vi "alum dose a+ b(HFTurbidity)0.5.vi"(4 "State":i16, 5 "Time":dbl format="%.2f", 6 "Sensor Values":dbl[](array[numeric]), 7 "Set Points":dbl[](array[numeric])) -> (0 "required data":T1={"Set Point names"=["a", "b", "raw water turbidity"], "required number of setpoints"=3, "required number of sensors"=0, "Sensor names"=[""]}, 3 "fraction on":dbl)   [LabVIEW 2010]
panel:
  # "Enter the correct information for this control code in the required data structure below. Then make the current value default by right clicking on the border of the data structure."
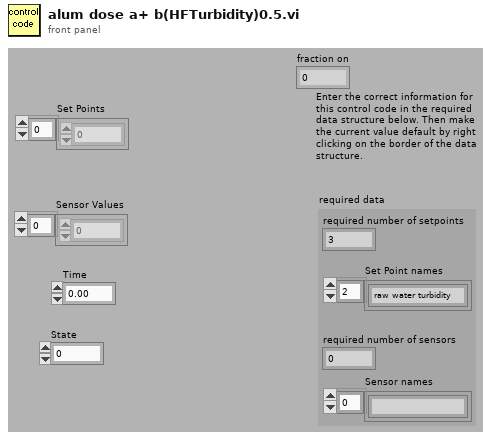
[diagram p1: front panel]
types:
  T1 = cluster{"Set Point names":string[], "required number of setpoints":u8, "required number of sensors":u8, "Sensor names":string[]}
  T2 = cluster{"Set Points[0]":dbl, "Set Points[1]":dbl, "Set Points[2]":dbl}
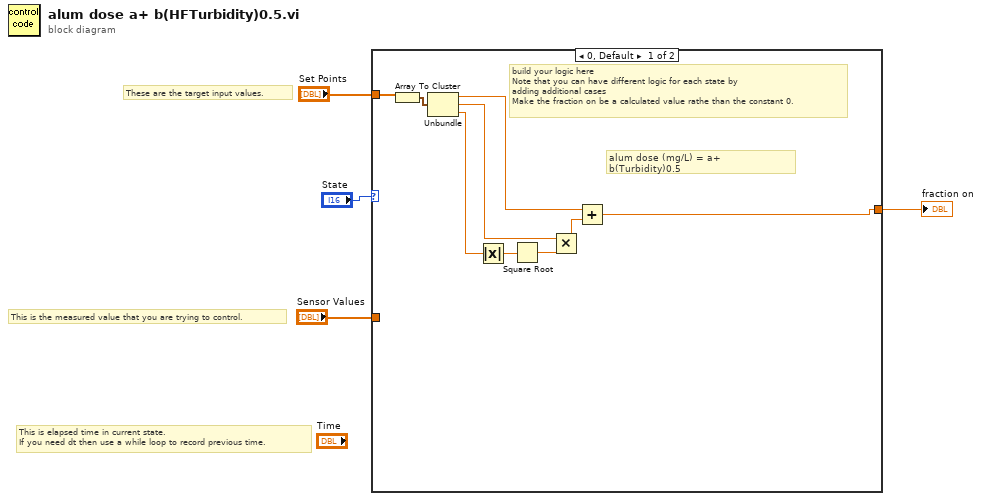
[diagram p0: block diagram]
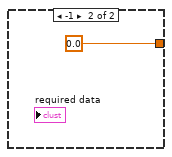
[diagram p2: hidden frame]
diagram:
  # "These are the target input values."
  # "This is the measured value that you are trying to control."
  # "This is elapsed time in current state.\nIf you need dt then use a while loop to record previous time."
  n1 = case shown="0, Default" "State" {
    tunnel: [w7 0.0 ("fraction on")] -> w3
    tunnel: "Set Points" -> [w13 _]
    tunnel: "Sensor Values" -> [_ _]
    frame 0, Default {
      # "alum dose (mg/L) = a+ b(Turbidity)0.5"
      # "build your logic here\nNote that you can have different logic for each state by\nadding additional cases\nMake the fraction on be a calculated value rathe than the constant 0."
      n2 = Array To Cluster(array=w13) -> (cluster=w12:T2)
      n3 = Unbundle(w12) -> ("Set Points[0]"=w9:dbl, "Set Points[1]"=w6:dbl, "Set Points[2]"=w5:dbl)
      n4 = Absolute Value(x=w5) -> (abs(x)=w11:dbl)
      n5 = Square Root(x=w11) -> (sqrt(x)=w10:dbl)
      n6 = Multiply(x=w6, y=w10) -> (x*y=w8:dbl)
      n7 = Add(x=w9, y=w8) -> (x+y=w7:dbl)
    }
    frame -1 {
    }
  }
  "fraction on" <- w3
